vi "DiffDriveKinematicsConstraint_getMinMaxAccel.vi"(8 "Velocity_M/S":dbl, 9 "Curvature":dbl, 10 "statePose":T4={"TRANSLATION"={"X"=0.0, "Y"=0.0}, "ROTATION"={"VALUE"=0.0, "COS"=1.0, "SIN"=0.0}} {"ROTATION"."SIN" format="%13.4f"; "ROTATION"."COS" format="%13.4f"; "ROTATION"."VALUE" format="%13.4f"; "TRANSLATION"."Y" format="%14.3f"; "TRANSLATION"."X" format="%14.3f"}, 11 "DIFF_DRIVE_KINE_CONSTRAINT":T1 {"Max Accel (M/S2)" format="%20.4f"; "DIFF_DRIVE_KINEMATICS"."TrackWidth_Meters" format="%20.4f"; "Max Speed (M/S)" format="%20.4f"}) -> (3 "TRAJ_CONSTAINT_MIN_MAX":T3)   [LabVIEW 2019, in "Trajectory_Library.lvlib"]
doc: "Return the minimum and maximum allowed acceleration given the provided conditions.\n\nIt appears that this routine doesn't do anything. It returns default values.\n\nParameters:\n - DiffDriveKinematicsConstraint - Constraint data structure\n - statePose - current traj state Pose\n - curvature - current traj curvature\n - maxVelocity - current traj max velocity\n\nReturns\n - TrajConstraint_Min_Max - Data structure with Min / Max acceleration."
uses:
  Trajectory_Library.lvlib
  POSE2D.ctl
  TRANSLATION2D.ctl
  ROTATION2D.ctl
  TRAJ_CONSTRAINT_MINMAX.ctl
  TRAJ_CONSTRAINT_DIIF_DRIVE_KINEMATICS.ctl
  DIFF_DRIVE_KINEMATICS.ctl
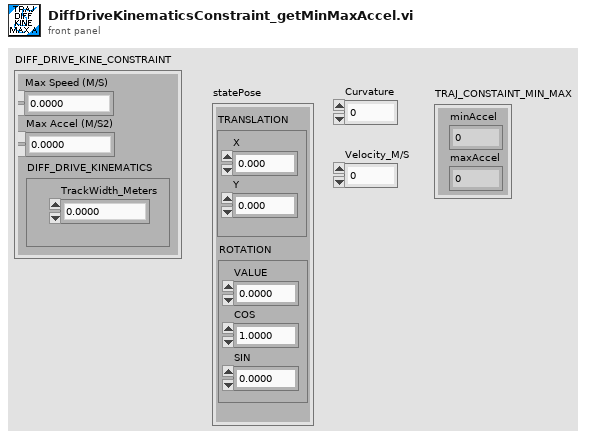
[diagram p1: front panel]
types:
  T1 = typedef "Trajectory_Library.lvlib/TRAJ_CONSTRAINT_DIIF_DRIVE_KINEMATICS.ctl" = cluster{"Max Speed (M/S)":dbl, "DIFF_DRIVE_KINEMATICS":T2, "Max Accel (M/S2)":dbl}
  T2 = typedef "Trajectory_Library.lvlib/DIFF_DRIVE_KINEMATICS.ctl" = cluster{"TrackWidth_Meters":dbl}
  T3 = typedef "Trajectory_Library.lvlib/TRAJ_CONSTRAINT_MINMAX.ctl" = cluster{"minAccel":dbl, "maxAccel":dbl}
  T4 = typedef "Trajectory_Library.lvlib/POSE2D.ctl" = cluster{"TRANSLATION":T5, "ROTATION":T6}
  T5 = typedef "Trajectory_Library.lvlib/TRANSLATION2D.ctl" = cluster{"X":dbl, "Y":dbl}
  T6 = typedef "Trajectory_Library.lvlib/ROTATION2D.ctl" = cluster{"VALUE":dbl, "COS":dbl, "SIN":dbl}
  T7 = typedef "Trajectory_Library.lvlib/CHASSIS_SPEEDS.ctl" = cluster{"vX":dbl, "vY":dbl, "vOmega":dbl}
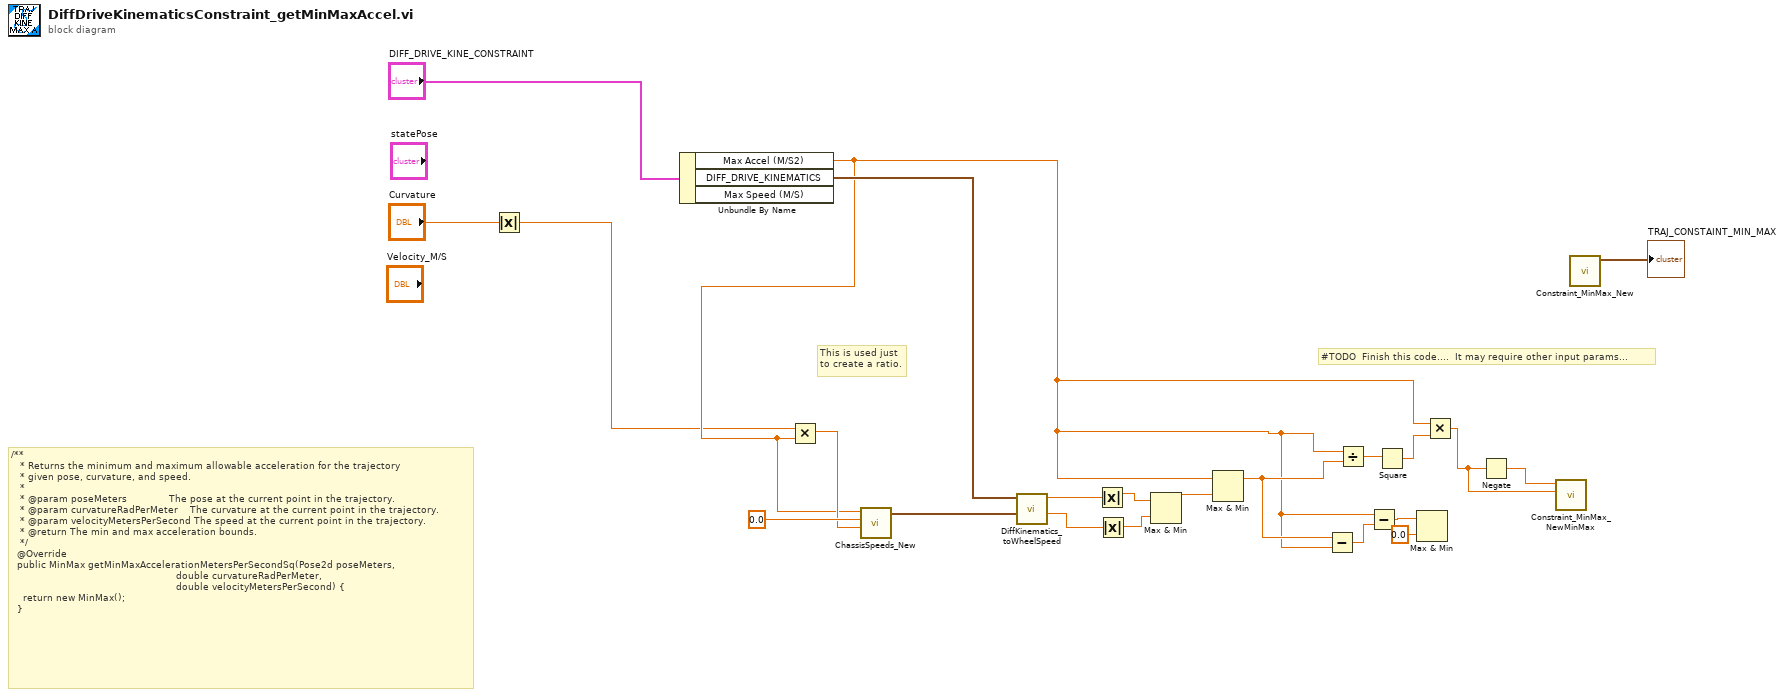
[diagram p0: block diagram]
diagram:
  # "#TODO  Finish this code....  It may require other input params..."
  # "This is used just\nto create a ratio."
  # "/**\n   * Returns the minimum and maximum allowable acceleration for the trajectory\n   * given pose, curvature, and speed.\n   *\n   * @param poseMeters              The pose at the current point in the trajectory.\n   * @param curvatureRadPerMeter    The curvature at the current point in the trajectory.\n   * @param velocityMetersPerSecond The speed at the current point in the trajectory.\n   * @return The min and max acceleration bounds.\n   */\n  @Override\n  public MinMax getMinMaxAccelerationMetersPerSecondSq(Pose2d poseMeters,\n                                                       double curvatureRadPerMeter,\n                                                       double velocityMetersPerSecond) {\n    return new MinMax();\n  }"
  n1 = Absolute Value(x="Curvature") -> (abs(x)=w4:dbl)
  n2 = Unbundle By Name("DIFF_DRIVE_KINE_CONSTRAINT") -> ("Max Accel (M/S2)"=w6:dbl, "DIFF_DRIVE_KINEMATICS"=w19:T2)  [unwired: 1 out]
  n3 = Multiply(x=w4, y=w6) -> (x*y=w21:dbl)
  n4 = call "ChassisSpeeds_New.vi"("vAngular"=w21, "vY"=0.0, "vX"=w6) -> ("CHASSIS"=w20:T7)  [unwired: 8 in]
  n5 = call "DiffKinematics_toWheelSpeed.vi"("CHASSIS Speed"=w20, "DIFF_DRIVE_KINEMATICS"=w19) -> ("RightVelocity"=w15:dbl, "LeftVelocity"=w16:dbl)  [unwired: 8 in]
  n6 = Absolute Value(x=w16) -> (abs(x)=w14:dbl)
  n7 = Absolute Value(x=w15) -> (abs(x)=w13:dbl)
  n8 = Max & Min(x=w14, y=w13) -> (max(x,y)=w12:dbl)  [unwired: 1 out]
  n9 = Max & Min(x=w6, y=w12) -> (max(x,y)=w11:dbl)  [unwired: 1 out]
  n10 = Subtract(x=w11, y=w6) -> (x-y=w10:dbl)
  n11 = Divide(x=w6, y=w11) -> (x/y=w3:dbl)
  n12 = Subtract(x=w6, y=w10) -> (x-y=w9:dbl)
  n13 = Square(x=w3) -> (x^2=w2:dbl)
  n14 = Max & Min(x=w9, y=0.0) -> ()  [unwired: 2 out]
  n15 = Multiply(x=w6, y=w2) -> (x*y=w5:dbl)
  n16 = Negate(x=w5) -> (-x=w17:dbl)
  n17 = call "Constraint_MinMax_NewMinMax.vi"("Max"=w5, "Min"=w17) -> ()  [unwired: 9 in, 1 out]
  n18 = call "Constraint_MinMax_New.vi"() -> ("TRAJ_CONSTAINT_MIN_MAX"=→"TRAJ_CONSTAINT_MIN_MAX":T3)  [unwired: 11 in]
